vi "startPlay.vi"(8 "error in (no error)":errorcluster, 11 "Football in":refnum<class "Football.lvclass">) -> (0 "error out":errorcluster, 3 "Football out":refnum<class "Football.lvclass">)   [LabVIEW 2017, in "Football.lvclass"]
uses:
  Football.lvclass
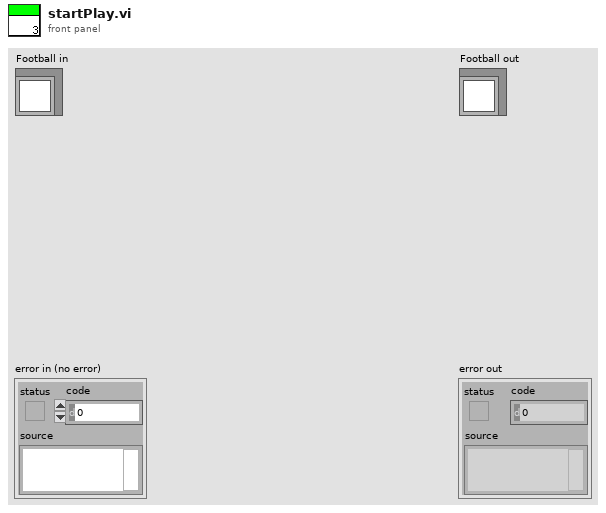
[diagram p1: front panel]
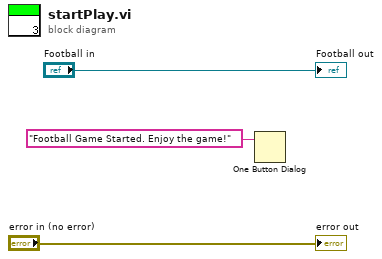
[diagram p0: block diagram]
diagram:
  n1 = One Button Dialog(message="Football Game Started. Enjoy the game!") -> ()  [unwired: 1 in, 1 out]
  "error out" <- "error in (no error)"
  "Football out" <- "Football in"
